vi "Periodic Tasks.vi"(8 "error in":errorcluster) -> ()   [LabVIEW 2016]
doc: "This VI runs in parallel to other tasks. It can contain as many user-defined periodic loops as you need. These can carry out PID or other sorts of timed response."
uses:
  Robot Global Data.vi
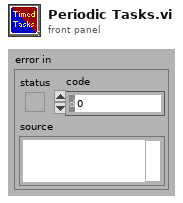
[diagram p1: front panel]
types:
  T1 = typedef "WPI_EncoderDevRef.ctl" = cluster{"DevStatus":errorcluster, "EncoderIndex":T2, "CounterIndex":T3, "DistancePerCount":dbl, "Decoding Type":T4}
  T2 = typedef "FPGA_EncoderIdx.ctl" = enum8{"Enc 0", "Enc 1", "Enc 2", "Enc 3", "Enc 4", "Enc 5", "Enc 6", "Enc 7", "Invalid"}
  T3 = typedef "FPGA_CounterCtrSystemIndex.ctl" = enum8{"Ctr 0", "Ctr 1", "Ctr 2", "Ctr 3", "Ctr 4", "Ctr 5", "Ctr 6", "Ctr 7", "Invalid"}
  T4 = typedef "WPI_EncoderType.ctl" = enum16{"1x", "2x", "4x"}
  T5 = typedef "WPI_DigitalInputDevRef.ctl" = cluster{"DevStatus":errorcluster, "DIO Channel":T6}
  T6 = typedef "FPGA_DIOChannel.ctl" = enum8{"DIO 0", "DIO 1", "DIO 2", "DIO 3", "DIO 4", "DIO 5", "DIO 6", "DIO 7", "DIO 8", "DIO 9", "DIO MXP 0", "DIO MXP 1", "DIO MXP 2", "DIO MXP 3", "DIO MXP 4", "DIO MXP 5", "DIO MXP 6", "DIO MXP 7", "DIO MXP 8", "DIO MXP 9", "DIO MXP 10", "DIO MXP 11", "DIO MXP 12", "DIO MXP 13", "DIO MXP 14", "DIO MXP 15", "SPI Port CS1", "SPI Port CS2", "SPI Port CS3", "SPI Port MISO", "SPI Port MOSI", "Invalid"}
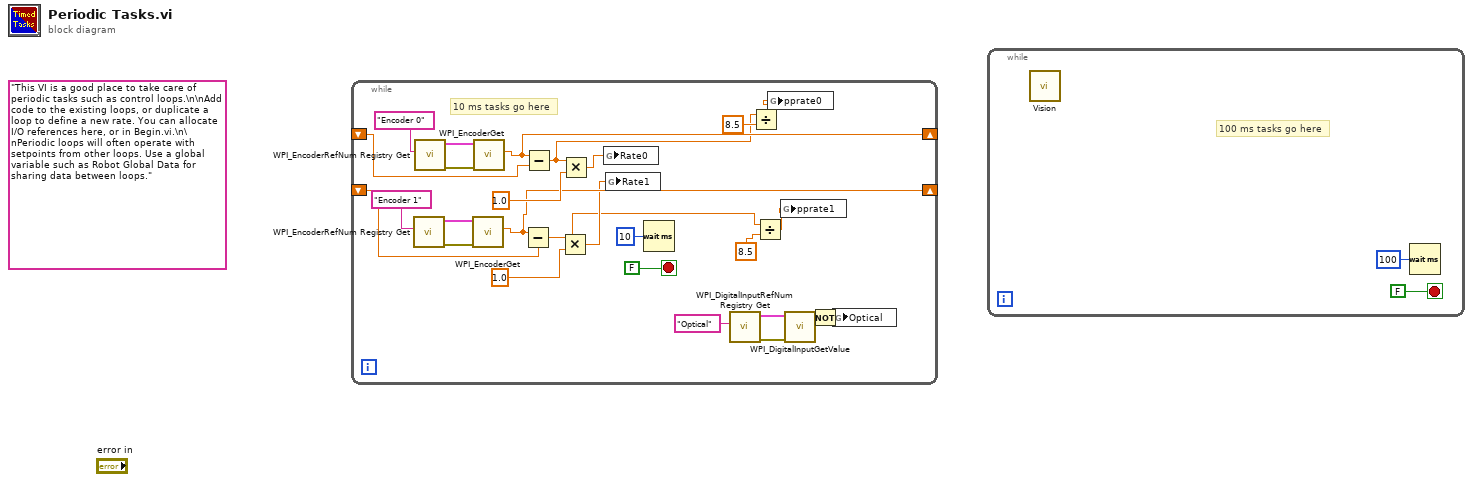
[diagram p0: block diagram]
diagram:
  (unwired) "This VI is a good place to take care of periodic tasks such as control loops.\n\nAdd code to the existing loops, or duplicate a loop to define a new rate. You can allocate I/O references here, or in Begin.vi.\n\nPeriodic loops will often operate with setpoints from other loops. Use a global variable such as Robot Global Data for sharing data between loops."
  n1 = while {
    shift-right: [w22] -> _
    shift-left: _ -> [w21]
    shift-right: [w14] -> _
    shift-left: _ -> [w15]
    stop <- FALSE stop-if-true
    # "10 ms tasks go here"
    n2 = call <vilib>:"WPI_EncoderRefNum Registry Get.vi"("refnum name"="Encoder 1") -> ("error out"=w19:errorcluster, "EncoderDevRef"=w18:T1)  [unwired: 9 in]
    n3 = call <vilib>:"WPI_EncoderRefNum Registry Get.vi"("refnum name"="Encoder 0") -> ("error out"=w25:errorcluster, "EncoderDevRef"=w24:T1)  [unwired: 9 in]
    n4 = call <vilib>:"WPI_EncoderGet.vi"("error in (no error)"=w19, "EncoderDevRef"=w18) -> ("Distance"=w14:dbl)  [unwired: 4 in, 5 out]
    n5 = call <vilib>:"WPI_EncoderGet.vi"("error in (no error)"=w25, "EncoderDevRef"=w24) -> ("Distance"=w22:dbl)  [unwired: 4 in, 5 out]
    n6 = Subtract(x=w14, y=w15) -> (x-y=w6:dbl)
    n7 = Subtract(x=w22, y=w21) -> (x-y=w7:dbl)
    n8 = Multiply(x=w6, y=1.0) -> (x*y=w12:dbl)
    n9 = Multiply(x=w7, y=1.0) -> (x*y=w13:dbl)
    n10 = global write "Robot Global Data.vi" "Rate0"(w13) -> ()
    n11 = global write "Robot Global Data.vi" "Rate1"(w12) -> ()
    n12 = Wait (ms)(milliseconds to wait=u32 10) -> ()  [unwired: 1 out]
    n13 = call <vilib>:"WPI_DigitalInputRefNum Registry Get.vi"("refnum name"="Optical") -> ("error out"=w5:errorcluster, "DigitalInputDevRef"=w4:T5)  [unwired: 9 in]
    n14 = Divide(x=w7, y=8.5) -> (x/y=w10:dbl)
    n15 = Divide(x=w6, y=8.5) -> (x/y=w11:dbl)
    n16 = global write "Robot Global Data.vi" "pprate0"(w10) -> ()
    n17 = global write "Robot Global Data.vi" "pprate1"(w11) -> ()
    n18 = call <vilib>:"WPI_DigitalInputGetValue.vi"("error in (no error)"=w5, "DigitalInputDevRef"=w4) -> ("Value"=w2:bool)  [unwired: 7 in, 2 out]
    n19 = Not(x=w2) -> (.not. x?=w1:bool)
    n20 = global write "Robot Global Data.vi" "Optical"(w1) -> ()
  }
  n21 = while {
    stop <- FALSE stop-if-true
    # "100 ms tasks go here"
    n22 = call "Vision.vi"() -> ()  [unwired: 12 in]
    n23 = Wait (ms)(milliseconds to wait=u32 100) -> ()  [unwired: 1 out]
  }
